vi "DigiPAC_COM_Check(SubVI).vi"(8 "error in (no error)":errorcluster, 9 "UART Channel (0)":u8, 11 "LINX Resource in":T1) -> (0 "error out":errorcluster, 1 "Confirmation message":string, 2 "Completed":bool, 3 "LINX Resource out":T1)   [LabVIEW 2017]
uses:
  <vilib>/MakerHub/LINX/Private/Type Defs/LINX Ref.ctl
  <vilib>/MakerHub/LINX/Private/Type Defs/Platform.ctl
  <vilib>/MakerHub/LINX/Private/Type Defs/Interface.ctl
  <vilib>/MakerHub/LINX/Private/Device/Type Defs/LINX Device Config.ctl
  <vilib>/MakerHub/LINX/Private/Device/Type Defs/TCP Config.ctl
  <vilib>/MakerHub/LINX/Private/Device/Type Defs/Channels.ctl
  <vilib>/MakerHub/LINX/Public/Peripherals/UART/UART Write String.vi
  <vilib>/MakerHub/LINX/Public/Peripherals/UART/UART Write Byte Array.vi
  <vilib>/MakerHub/LINX/Private/Local IO/LinxUartWrite.vi
  <vilib>/MakerHub/LINX/Public/Utilities/Check Channel.vi
  <vilib>/MakerHub/LINX/Private/Utilties/Generate Error.vi
  <vilib>/MakerHub/LINX/Public/Peripherals/UART/UART Read String.vi
  <vilib>/MakerHub/LINX/LMH-LINX.lvlib
  <vilib>/MakerHub/LINX/Private/Device/Device.lvlib
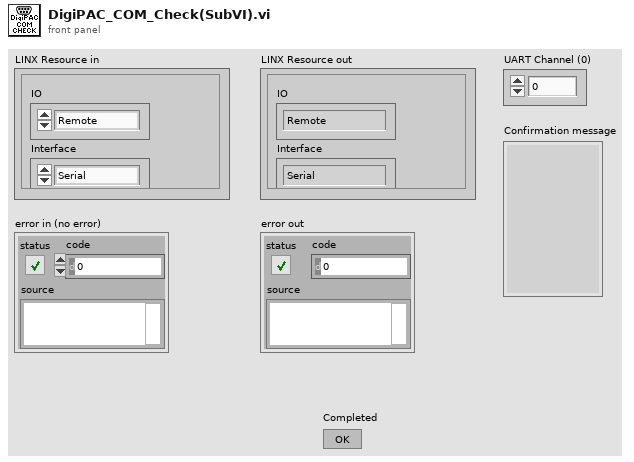
[diagram p1: front panel]
types:
  T1 = typedef "LMH-LINX.lvlib/LINX Ref.ctl" = cluster{"IO":T2, "Interface":T3, "LINX Device Config":T4}
  T2 = typedef "LMH-LINX.lvlib/Platform.ctl" = enum16{"Remote", "Local"}
  T3 = typedef "LMH-LINX.lvlib/Interface.ctl" = enum16{"Serial", "TCP"}
  T4 = typedef "LMH-LINX.lvlib/Device.lvlib/LINX Device Config.ctl" = cluster{"Interface":T3, "COM Port":refnum<visa-resource-name>, "TCP Configuration":T5, "Device Family":u8, "Device ID":u8, "Device Name":string, "TCP Ref":refnum<k5>, "Channels":T6}
  T5 = typedef "LMH-LINX.lvlib/Device.lvlib/TCP Config.ctl" = cluster{"IP Address":string, "Port":u16}
  T6 = typedef "LMH-LINX.lvlib/Channels.ctl" = cluster{"DI":u8[], "DO":u8[], "AI":u8[], "AO":u8[], "PWM":u8[], "QE":u8[], "UART":u8[], "I2C 2":u8[], "SPI":u8[], "CAN":u8[], "Servo":u8[], "AI Ref (V)":dbl, "AI Resolution (Bits)":u8, "AO Ref (V)":dbl, "AO Resolution (Bits)":u8}
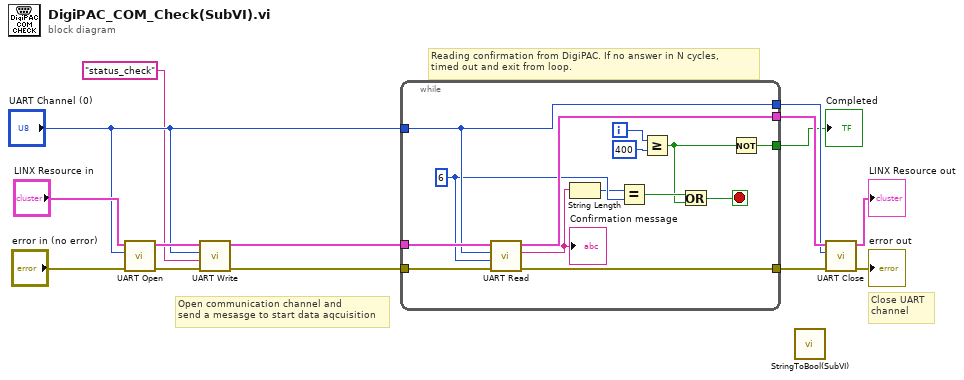
[diagram p0: block diagram]
diagram:
  # "Close UART\nchannel"
  # "Open communication channel and \nsend a mesasge to start data aqcuisition"
  # "Reading confirmation from DigiPAC. If no answer in N cycles, \ntimed out and exit from loop."
  n1 = call <vilib>:"UART Open.vi"("Error In"="error in (no error)", "UART Channel (0)"="UART Channel (0)", "LINX Resource"="LINX Resource in") -> ("Error Out"=w11:errorcluster, "LINX Resource"=w12:T1)  [unwired: 6 in, 1 out]
  n2 = call-poly <vilib>:"UART Write.vi"("Error In"=w11, "Data"="status_check", "UART Channel (0)"="UART Channel (0)", "LINX Resource"=w12) -> ("Error Out"=w9:errorcluster, "LINX Resource"=w10:T1)  [unwired: 6 in]
  n3 = while {
    tunnel: w10 -> [w28]
    tunnel: w9 -> [w27]
    tunnel: [w26] -> w8
    tunnel: [w25] -> w7
    tunnel: "UART Channel (0)" -> [w24]
    tunnel: [w24] -> w6
    tunnel: [w18] -> w2
    i -> [w23]
    stop <- w20 stop-if-true
    w17 = u8 6 ("Num Bytes")
    n4 = call-poly <vilib>:"UART Read.vi"("Error In"=w27, "Num Bytes"=w17, "UART Channel (0)"=w24, "LINX Resource"=w28) -> ("Error Out"=w25:errorcluster, "Data"=w15:string, "LINX Resource"=w26:T1)  [unwired: 5 in]
    "Confirmation message" <- w15
    n5 = String Length(string=w15) -> (length=w16:i32)
    n6 = Equal?(x=w16, y=w17) -> (x = y?=w21:bool)
    n7 = Greater Or Equal?(x=w23, y=400) -> (x >= y?=w19:bool)
    n8 = Or(x=w21, y=w19) -> (x .or. y?=w20:bool)
    n9 = Not(x=w19) -> (.not. x?=w18:bool)
  }
  "Completed" <- w2
  n10 = call "StringToBool(SubVI).vi"() -> ()  [unwired: 5 in, 6 out]
  n11 = call <vilib>:"UART Close.vi"("Error In"=w7, "UART Channel (0)"=w6, "LINX Resource"=w8) -> ("Error Out"=→"error out":errorcluster, "LINX Resource"=→"LINX Resource out":T1)  [unwired: 7 in]
